vi "Configure Event Search (Serial Bus - I2S).vi"(4 "Qualifier (0: Equal)":i32(ring) items=["Equal", "Not Equal", "Less", "Greater", "In Range", "Out Range"], 5 "Data Low Limit (-10)":i32=-10, 6 "Data High Limit (10)":i32=10, 7 "Data Format (2: Decimal)":i32(ring)=2 items=["Binary", "Hex", "Decimal"], 8 "error in (no error)":errorcluster, 9 "Data Value (0)":string="0", 10 "Source Channel (0: Right Channel)":i32(ring) items=["Right Channel", "Left Channel", "Either Channel"], 11 "VISA resource name":refnum<visa-resource-name>) -> (0 "error out":errorcluster, 3 "VISA resource name out":refnum<visa-resource-name>)   [LabVIEW 2023, in "Keysight-DSQx3014T.lvlib"]
doc: "Configures the event search of I2S bus."
uses:
  Keysight-DSQx3014T.lvlib
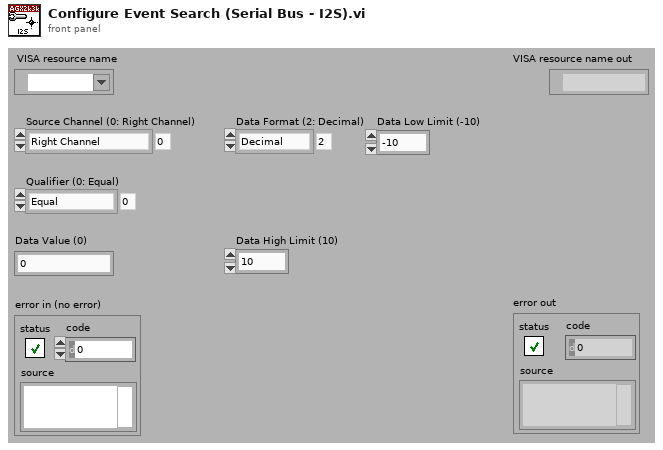
[diagram p1: front panel]
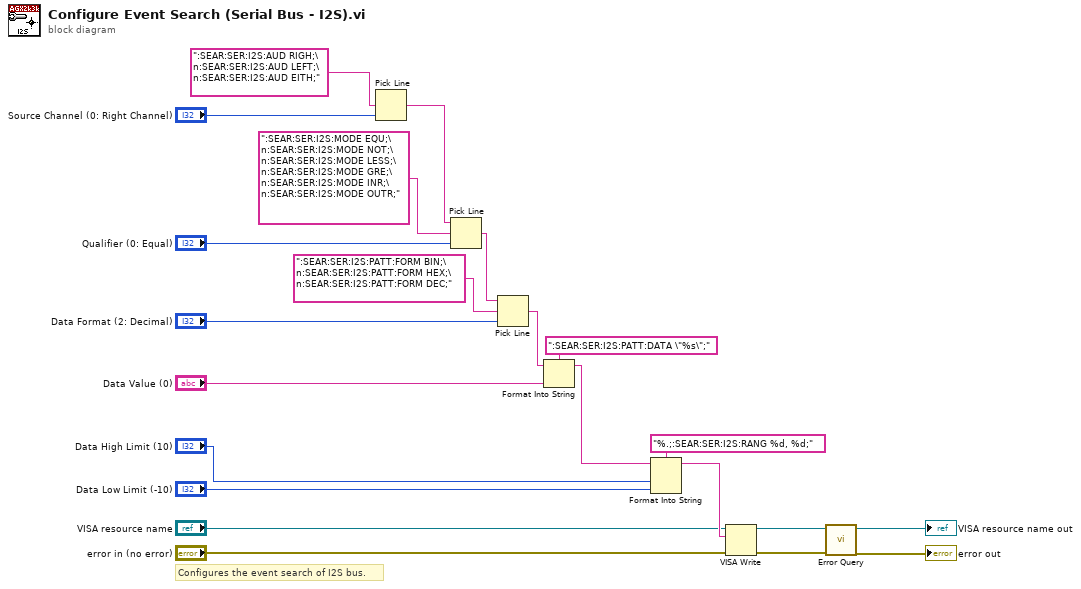
[diagram p0: block diagram]
diagram:
  # "Configures the event search of I2S bus."
  n1 = Pick Line(multi-line string=":SEAR:SER:I2S:AUD RIGH;\n:SEAR:SER:I2S:AUD LEFT;\n:SEAR:SER:I2S:AUD EITH;", line index="Source Channel (0: Right Channel)") -> (output string=w18:string)  [unwired: 1 out]
  n2 = Pick Line(string ("")=w18, multi-line string=":SEAR:SER:I2S:MODE EQU;\n:SEAR:SER:I2S:MODE NOT;\n:SEAR:SER:I2S:MODE LESS;\n:SEAR:SER:I2S:MODE GRE;\n:SEAR:SER:I2S:MODE INR;\n:SEAR:SER:I2S:MODE OUTR;", line index="Qualifier (0: Equal)") -> (output string=w3:string)
  n3 = Pick Line(string ("")=w3, multi-line string=":SEAR:SER:I2S:PATT:FORM BIN;\n:SEAR:SER:I2S:PATT:FORM HEX;\n:SEAR:SER:I2S:PATT:FORM DEC;", line index="Data Format (2: Decimal)") -> (output string=w2:string)
  n4 = Format Into String(format string=":SEAR:SER:I2S:PATT:DATA \"%s\";", initial string=w2, "Data Value (0)") -> (resulting string=w1:string)  [unwired: 1 in, 1 out]
  n5 = Format Into String(format string="%.;:SEAR:SER:I2S:RANG %d, %d;", initial string=w1, "Data High Limit (10)", "Data Low Limit (-10)") -> (resulting string=w10:string)  [unwired: 1 in, 1 out]
  n6 = VISA Write(VISA resource name="VISA resource name", write buffer=w10, error in (no error)="error in (no error)") -> (VISA resource name out=w7:refnum<visa-resource-name>, error out=w6:errorcluster)  [unwired: 1 out]
  n7 = call "Error Query.vi"("error in (no error)"=w6, "VISA resource name"=w7) -> ("error out"=→"error out":errorcluster, "VISA resource name out"=→"VISA resource name out":refnum<visa-resource-name>)  [unwired: 8 out]
